vi "Rms (SubVI).vi"(1 "Fs":dbl, 2 "Array":dbl[](array[numeric])) -> (0 "Y":dbl[](array[numeric]))   [LabVIEW 2014]
uses:
  <vilib>/addons/Sound and Vibration/svt_Weighting/SVT A, B, C Weighting Filter (Fixed Rates) (1 Ch).vi
  <vilib>/addons/Sound and Vibration/svt_Level/SVL Exp Avg Sound Level (1 Ch).vi
  <vilib>/addons/Sound and Vibration/svt_Level/SoundVib_SoundLevel.lvlib
  <vilib>/addons/Sound and Vibration/svt_Weighting/SoundVib_ABCWeighting.lvlib
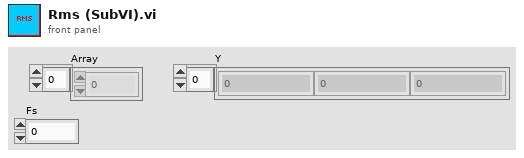
[diagram p1: front panel]
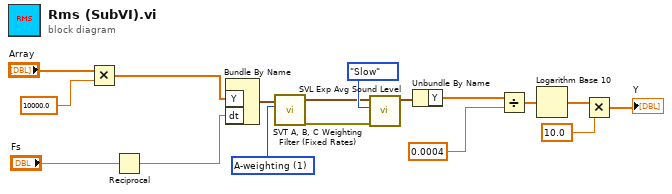
[diagram p0: block diagram]
diagram:
  w16 = u16 1 items=["Linear", "A-weighting", "B-weighting", "C-weighting"] ("weighting")
  n1 = Multiply(x="Array", y=10000.0) -> (x*y=w7:dbl[])
  n2 = Reciprocal(x="Fs") -> (1/x=w11:dbl)
  n3 = Bundle By Name("Y"=w7, "dt"=w11) -> (w12:waveform(dbl))  [unwired: 1 in]
  n4 = call-poly <vilib>:"SVT A, B, C Weighting Filter (Fixed Rates).vi"("weighting"=w16, "scaled signal [EU]"=w12) -> ("error out"=w15:errorcluster, "weighted signal [EU]"=w14:waveform(dbl))  [unwired: 7 in]
  n5 = call-poly <vilib>:"SVL Exp Avg Sound Level.vi"("error in (no error)"=w15, "exponential mode"=enum16{"Slow", "Fast", "Impulse", "Custom"}."Slow", "scaled signal [EU]"=w14) -> ("exp avg sound level [dB EU]"=w13:waveform(dbl))  [unwired: 4 in, 4 out]
  n6 = Unbundle By Name(w13) -> ("Y"=w3:dbl[])
  n7 = Divide(x=w3, y=0.0004) -> (x/y=w4:dbl[])
  n8 = Logarithm Base 10(1:w4) -> (0:w5:dbl[])
  n9 = Multiply(x=w5, y=10.0) -> (x*y=→"Y":dbl[])
